vi "get faults.vi"(8 "error in (no error)":errorcluster, 11 "Cobolt in":refnum<class "Cobolt.lvclass">) -> (0 "error out":errorcluster, 3 "Cobolt out":refnum<class "Cobolt.lvclass">)   [LabVIEW 2012, in "Cobolt.lvclass"]
uses:
  Cobolt.lvclass
  CoboltLaserDrivers_Public_LV2012/CoboltLaser_Controls/ExpectedResponseType.ctl
  Cobolt.lvclass/Cobolt.ctl
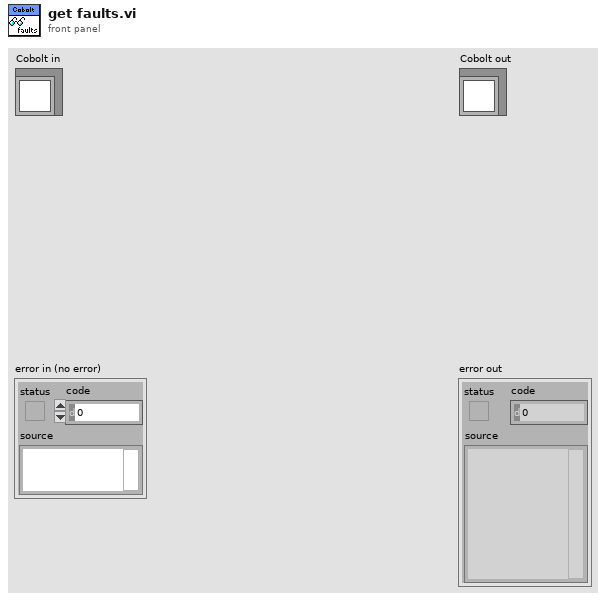
[diagram p1: front panel]
types:
  T1 = typedef "Cobolt.lvclass/ExpectedResponseType.ctl" = u16
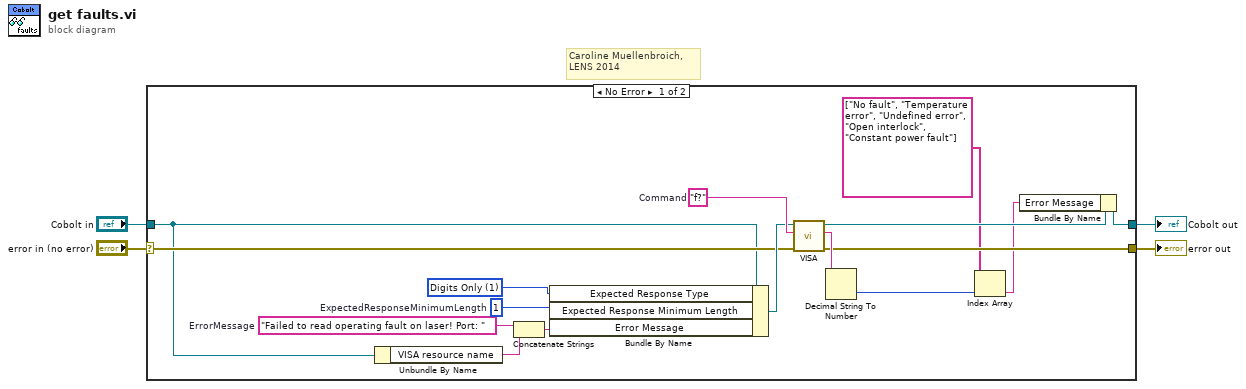
[diagram p0: block diagram]
diagram:
  # "Caroline Muellenbroich, \nLENS 2014"
  n1 = case shown="No Error" "error in (no error)" {
    selector: "error in (no error)" -> [w11 w22]
    tunnel: [w10 w22] -> w3
    tunnel: [w8 w21] -> w1
    tunnel: "Cobolt in" -> [w9 w21]
    frame No Error {
      w13 = T1 1 items=["Any", "Digits Only", "Non-Digits Only"] ("ExpectedResponseType")
      w17 = 1  # ExpectedResponseMinimumLength
      w15 = "Failed to read operating fault on laser! Port: "  # ErrorMessage
      w19 = "f?"  # Command
      n2 = Unbundle By Name(w9) -> ("VISA resource name"=w16:string)
      n3 = Concatenate Strings(w15, w16) -> (w14:string)
      n4 = Bundle By Name(cluster=w9, "Expected Response Type"=w13, "Expected Response Minimum Length"=w17, "Error Message"=w14) -> (w18:refnum<class "Cobolt.lvclass">)
      n5 = call-dynamic "VISA.vi"("error in (no error)"=w11, "string to write"=w19, "Cobolt in"=w18) -> ("error out"=w10:errorcluster, "buffer out"=w12:string, "Cobolt out"=w20:refnum<class "Cobolt.lvclass">)  [unwired: 6 in]
      n6 = Decimal String To Number(string=w12) -> (number=w7:i32)  [unwired: 2 in, 1 out]
      n7 = Index Array(array=string[] ["No fault", "Temperature error", "Undefined error", "Open interlock", "Constant power fault"], index=w7) -> (element=w5:string)
      n8 = Bundle By Name(cluster=w20, "Error Message"=w5) -> (w8:refnum<class "Cobolt.lvclass">)
    }
    frame Error {
    }
  }
  "error out" <- w3
  "Cobolt out" <- w1
